vi "Read Gantry Driver.vi"(8 "error in (no error)":errorcluster, 11 "Gantry in":refnum<class "Gantry.lvclass">) -> (0 "error out":errorcluster, 2 "Gantry Driver":T1, 3 "Gantry out":refnum<class "Gantry.lvclass">)   [LabVIEW 2024, in "Gantry.lvclass"]
uses:
  Gantry.lvclass
  Gantry.lvclass/Gantry.ctl
  Type Definitions/Gantry Driver.ctl
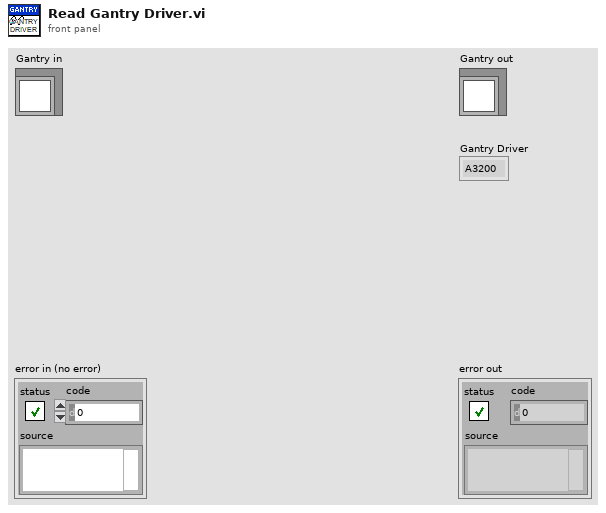
[diagram p1: front panel]
types:
  T1 = typedef "Gantry Driver.ctl" = enum16{"A3200", "AUTOMATION1", "VIRTUAL"}
  T2 = typedef "Virtual Modes.ctl" = enum16{"Nonvirtual", "Virtual"}
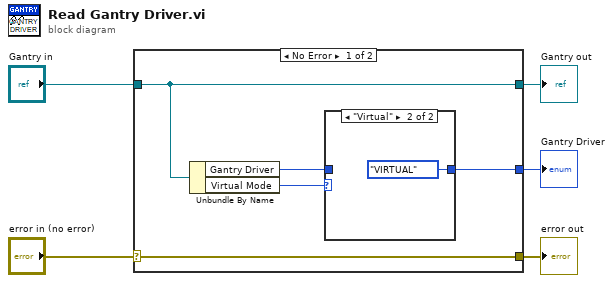
[diagram p0: block diagram]
diagram:
  n1 = case shown="No Error" "error in (no error)" {
    selector: "error in (no error)" -> [w10 w13]
    tunnel: [w10 w13] -> w4
    tunnel: [w9 w14] -> w2
    tunnel: "Gantry in" -> [w9 w14]
    tunnel: [w6 _] -> w1
    frame No Error {
      n2 = Unbundle By Name(w9) -> ("Gantry Driver"=w7:T1, "Virtual Mode"=w8:T2)
      n3 = case shown="\"Virtual\"" w8 {
        tunnel: w7 -> [w11 _]
        tunnel: [w11 Gantry_Driver."VIRTUAL" ("Gantry Driver")] -> w6
        frame "Nonvirtual", Default {
        }
        frame "Virtual" {
        }
      }
    }
    frame Error {
    }
  }
  "error out" <- w4
  "Gantry out" <- w2
  "Gantry Driver" <- w1
